vi "Record_global.vi"() -> ()   [LabVIEW 2014]
panel:
  in  "Cycle":string
  in  "Record":bool
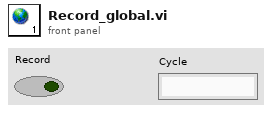
[diagram p1: front panel]
diagram:
